vi "PH_Beamline.ProcEvents.vi"(0 "i ref in":refnum<vi>, 5 "error in (no error)":errorcluster) -> (14 "i ref out":refnum<vi>, 19 "error out":errorcluster)   [LabVIEW 2014, in "PH_Beamline.lvlib"]
doc: "This method is used to define the events the object will listen to. Add your own events here."
uses:
  PH_Beamline.lvlib
  CSCore/BaseProcess/BaseProcess.lvlib
  PH_Common/PH_Common.lvlib
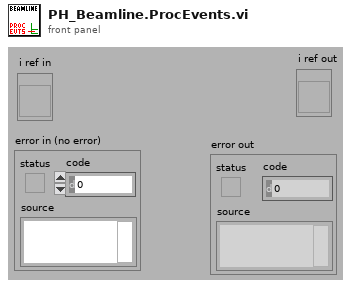
[diagram p1: front panel]
types:
  T1 = typedef "PH_Beamline.lvlib/PH_Beamline.i attribute.ctl" = cluster{"GUI Refs":cluster{"PA ok":refnum<vi>, "MA ok":refnum<vi>, "fs FE ok":refnum<vi>, "ns FE ok":refnum<vi>, "PA ED ok":refnum<vi>, "MAS ok":refnum<vi>, "Booster ok":refnum<vi>, "Mirrortower ok":refnum<vi>, "In.-Box ok":refnum<vi>, "Compressor ok":refnum<vi>, "Experiment LB ok":refnum<vi>, "Experiment LL ok":refnum<vi>, "PHELIX_Beckhoff_Watchdog":refnum<vi>, "Shutters closed":refnum<vi>, "uOPA ok":refnum<vi>, "Vacuum no shotcond Comp LB":refnum<vi>}, "Refs BL MA":refnum<vi>[], "Refs BL MA-IB":refnum<vi>[], "Refs BL fs":refnum<vi>[], "Refs BL PA ED":refnum<vi>[], "Refs BL MAS":refnum<vi>[], "Refs BL Boo":refnum<vi>[], "Refs BL ns":refnum<vi>[], "Refs BL Mirrortower":refnum<vi>[], "Refs BL Compressor":refnum<vi>[], "Refs BL Exp LB":refnum<vi>[], "Radiation Safety":cluster{"Exp Laserbay":cluster{"Ref Op Mode":refnum<vi>, "Ref Laserbay evacuated":refnum<vi>, "Tagname LB evacuated":string, "Shot Mode":T2, "Laserbay evacuated?":i32, "Tagname HV room locked":string, "HV room locked?":i32, "Ref HV room locked":refnum<vi>, "Tagname bridged?":string, "Ref Bridge":refnum<vi>, "I<1E18W/cm²":bool}, "Exp Laserlab":cluster{"Ref Op Mode":refnum<vi>, "Ref Laserlab evacuated":refnum<vi>, "Tagname LL evacuated":string, "Shot Mode":T2, "Laserlab evacuated?":i32, "Tagname bridged?":string, "Ref Bridge":refnum<vi>, "I<1E18W/cm²":bool}}, "Refs BL LL":refnum<vi>[], "PP Igni Heating GUI Refs":refnum<vi>[], "PP Igni Heating Tagnames ":string[], "Refs BL PA":cluster{"undelayed Line before Shutter":refnum<vi>[], "undelayed Line after Shutter":refnum<vi>[], "before Bypass":refnum<vi>[], "delayed Line before Shutter":refnum<vi>[], "delayed Line after Shutter":refnum<vi>[], "before Shutter Input":refnum<vi>[], "after Shutter Input":refnum<vi>[], "Bypass":refnum<vi>[], "before Shutter Exit":refnum<vi>[], "after Shutter Exit":refnum<vi>[], "to MA":refnum<vi>[], "to Lab":refnum<vi>[]}, "BL":cluster{"YLF_BL_Status":i32, "fs_BL_Status":i32, "fs_YLF_BL_Status":i32, "ns_BL_Status":i32, "PA_Input_BL_Status":i32, "PA_UnDelay_BL_Status":i32, "PA_Delay_BL_Status":i32, "PA_BL_Status":i32, "PA_Bypass_BL_Status":i32, "PA_Exit_BL_Status":i32, "PA_LL_BL_Status":i32, "LL_BL_Status":i32, "PA_MA_BL_Status":i32, "MA_Exit_BL_Status":i32, "MA_Z6_BL_Status":i32, "Z6_BL_Status":i32, "MA_LB_BL_Status":i32, "LB_TB2_BL_Status":i32, "PA_before_Bypass_BL_Status":i32, "LB_TB3_BL_Status":i32}, "State Subsystems":cluster{"PA":bool, "MA":bool, "ns FE":bool, "fs FE":bool, "PA ED":bool, "In.-Box":bool, "MAS":bool, "Booster":bool, "Mirrortower":bool, "Compressor":bool, "Experiment LB":bool, "Experiment LL":bool, "uOPA":bool}, "Status Subscriber Information":T3, "Refs BL uOPA":refnum<vi>[], "PA_Input_2_Beam_6PWpGUI not linked?":bool, "PA_Input_Delay_6PGUI not linked?":bool, "Settings":T6}
  T2 = typedef "PH_Beamline.lvlib/PH_Beamline.Operation Mode.ctl" = i32
  T3 = typedef "PH_Beamline.lvlib/PH_Beamline.Status Subscriber Information.ctl" = cluster{"fs Swich YLF":T4, "fs Exit Shutter":T4, "ns Exit Shutter":T4, "PA Input Shutter":T4, "PA PC WP":T4, "PA PC WP 2":T4, "PA Bypass In":T4, "PA Bypass Out":T4, "PA CH 1":T4, "PA delayed":T4, "PA non delayed":T4, "PA Exit Shutter":T4, "PA Switch Lab":T4, "PA Bridge CH Input MA":T4, "MA Diffusor IB":T4, "MA IB Ready":T4, "MA CH 1":T4, "MA CH 2":T4, "MA CH 3":T4, "MA CH 4":T4, "MA Shutter Align Cam":T4, "MA Position MM5":T4, "Calorimeter Switch":T4, "BL Z6 CH 9":T4, "BL Z6 Beamdump":T4, "BL Z6 Shutter":T4, "COS Sensitivity Switch":T4, "Exp LB Shutter":T4, "Exp LB TB 2":T4, "Exp LB TB 3":T4, "PA LL Input CH":T4, "PA LL Output CH":T4, "LL Comp Input Shutter":T4, "LL Comp Output Shutter":T4, "LL Comp FF Shutter":T4, "Exp LL Shutter":T4, "MA IM In IB":T4, "MA IM Out IB":T4, "MA DB In IB":T4, "MA DB Out IB":T4, "Exp LB Shutter Interlock":T4, "Exp LL Shutter Interlock":T4, "MM1 Force Sensor":T4}
  T4 = typedef "PH_BL-Master.lvlib/PH_BL-Master.Status Subscriber Information.ctl" = cluster{"Index of element":i32, "Attributeset":T5}
  T5 = typedef "PH_BL-Master.lvlib/PH_BL-Master.Attribute Set.ctl" = enum16{"Boolean Status Service Subscriber", "Picture Status Service Subscriber"}
  T6 = typedef "PH_Beamline_Chief.lvlib/PH_Beamline_Chief.Settings.ctl" = cluster{"PA Doublepass Mode":bool, "Compressor Vaccuum LB not relevant":bool, "Windowshutter TB2 not relevant":bool, "Windowshutter TB3 not relevant":bool}
  T7 = typedef "PH_Common.lvlib/PH_DIM.Event Declarer.ctl" = cluster{"Service Name":string, "Selector":string}
  T8 = typedef "BaseProcess.lvlib/BaseProcess.event definition.ctl" = cluster{"CAEEvtDef":T9, "Data Descriptor":T10}
  T9 = typedef "CAEObj.lvlib/CAEObj.event definition.ctl" = cluster{"URL":string, "enable":bool, "ignoreResID":bool}
  T10 = typedef "BaseProcess.lvlib/BaseProcess.descriptor string definition.ctl" = string
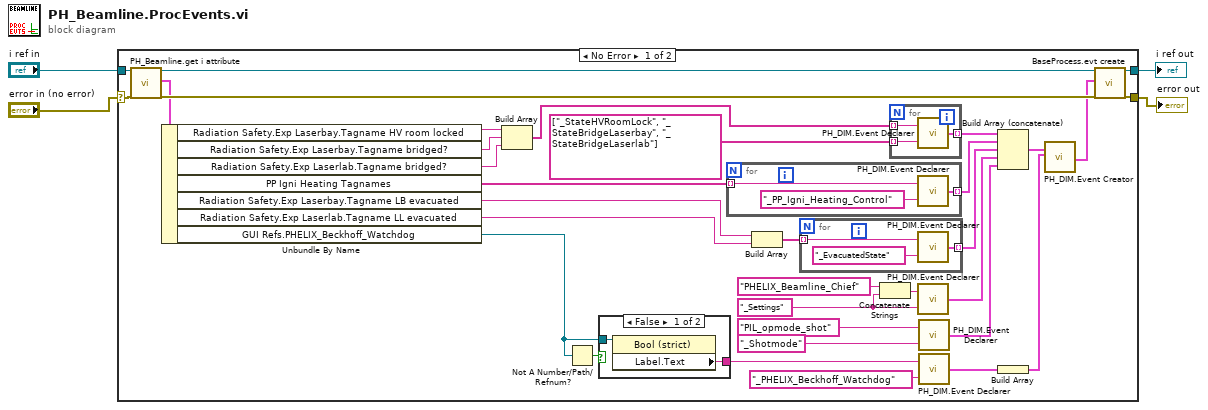
[diagram p0: block diagram]
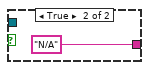
[diagram p2: hidden frame]
diagram:
  n1 = case shown="No Error" "error in (no error)" {
    selector: "error in (no error)" -> [w32 w51]
    tunnel: [w38 w51] -> w4
    tunnel: [w37 w52] -> w3
    tunnel: "i ref in" -> [w36 w52]
    frame No Error {
      w13 = "_Settings"
      n2 = call "PH_Beamline.get i attribute.vi"("i ref in"=w36, "error in (no error)"=w32) -> ("i ref out"=w35:refnum<vi>, "i attribute"=w33:T1, "error out"=w34:errorcluster)  [unwired: 15 in]
      n3 = Unbundle By Name(w33) -> ("Radiation Safety.Exp Laserbay.Tagname HV room locked"=w22:string, "Radiation Safety.Exp Laserbay.Tagname bridged?"=w21:string, "Radiation Safety.Exp Laserlab.Tagname bridged?"=w20:string, "PP Igni Heating Tagnames"=w30:string[], "Radiation Safety.Exp Laserbay.Tagname LB evacuated"=w28:string, "Radiation Safety.Exp Laserlab.Tagname LL evacuated"=w27:string, "GUI Refs.PHELIX_Beckhoff_Watchdog"=w23:refnum<vi>)
      n4 = Build Array(w22, w21, w20) -> (w17:string[])
      n5 = Not A Number/Path/Refnum?(number/path/refnum=w23) -> (NaN/Path/Refnum?=w24:bool)
      n6 = case shown="False" w24 {
        tunnel: w23 -> [w43 _]
        tunnel: [w42 "N/A" ("Label.Text")] -> w15
        frame False {
          n7 = property class="Bool (strict)"(reference=w43) -> ("Label.Text"=w42:string)  [unwired: 1 in, 2 out]
        }
        frame True {
        }
      }
      n8 = for {
        tunnel: [w49] -> w29 mode=indexing
        tunnel: w30 -> [w48] mode=indexing
        n9 = call "PH_DIM.Event Declarer.vi"("Selector"="_PP_Igni_Heating_Control", "Service Name"=w48) -> ("declared DIM Event"=w49:T7)
      }
      n10 = Build Array(w28, w27) -> (w26:string[])
      n11 = for {
        tunnel: [w46] -> w25 mode=indexing
        tunnel: w26 -> [w45] mode=indexing
        n12 = call "PH_DIM.Event Declarer.vi"("Selector"="_EvacuatedState", "Service Name"=w45) -> ("declared DIM Event"=w46:T7)
      }
      n13 = Concatenate Strings("PHELIX_Beamline_Chief" ("string"), w13) -> (w14:string)
      n14 = for {
        tunnel: [w41] -> w19 mode=indexing
        tunnel: w17 -> [w40] mode=indexing
        tunnel: string[] ["_StateHVRoomLock", "_StateBridgeLaserbay", "_StateBridgeLaserlab"] -> [w39] mode=indexing
        n15 = call "PH_DIM.Event Declarer.vi"("Selector"=w39, "Service Name"=w40) -> ("declared DIM Event"=w41:T7)
      }
      n16 = call "PH_DIM.Event Declarer.vi"("Selector"=w13, "Service Name"=w14) -> ("declared DIM Event"=w11:T7)
      n17 = call "PH_DIM.Event Declarer.vi"("Selector"="_Shotmode", "Service Name"="PIL_opmode_shot") -> ("declared DIM Event"=w6:T7)
      n18 = call "PH_DIM.Event Declarer.vi"("Selector"="_PHELIX_Beckhoff_Watchdog", "Service Name"=w15) -> ("declared DIM Event"=w16:T7)
      n19 = Build Array (concatenate)(w19, w29, w25, w11, w6) -> (w31:T7[])
      n20 = Build Array(w16) -> (w9:T7[])
      n21 = call "PH_DIM.Event Creator.vi"("Trendmessage Services"=w31, "Status Services"=w9) -> ("DIM Service Events"=w5:T8[])  [unwired: 17 in]
      n22 = call "BaseProcess.evt create.vi"("i ref in"=w35, "newEvents"=w5, "error in (no error)"=w34) -> ("i ref out"=w37:refnum<vi>, "error out"=w38:errorcluster)  [unwired: 13 in, 2 out]
    }
    frame Error {
    }
  }
  "i ref out" <- w3
  "error out" <- w4
